vi "LCfiletrans(SubVI).vi"(8 "error in (no error)":errorcluster, 9 "Source Filename":string="D:\\Automation\\Data\\C1Title00030.csv", 11 "VISA Refnum in":refnum<visa-resource-name>="LecroyHDO4024-1") -> (0 "error out":errorcluster, 2 "File data":string, 3 "VISA Refnum out":refnum<visa-resource-name>)   [LabVIEW 2018]
uses:
  <instrlib>/LeCroy Wave Series/LeCroy Wave Series.lvlib
panel:
  in  "file path (use dialog)":path=path "E:/Ankur/Labview/Automation/Files/Oscdata/C1Title00030.csv"
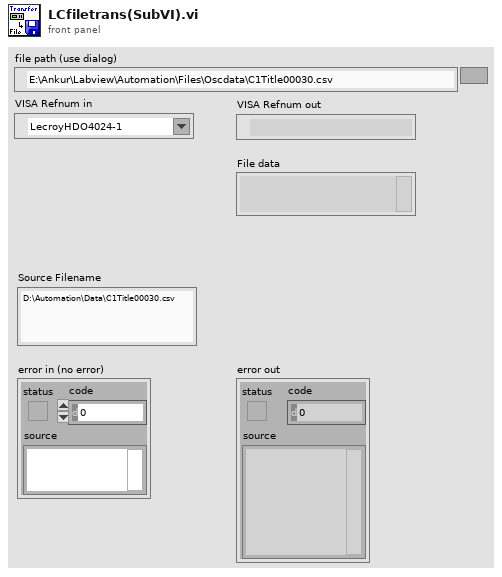
[diagram p1: front panel]
types:
  T1 = enum16{"open", "replace", "create", "open or create", "replace or create", "replace or create with confirmation"}
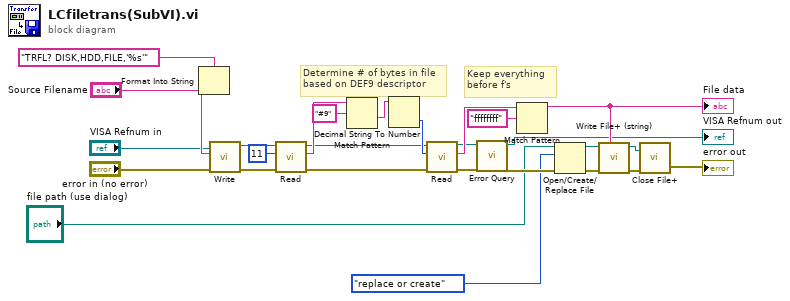
[diagram p0: block diagram]
diagram:
  # "Keep everything \nbefore f's"
  # "Determine # of bytes in file\nbased on DEF9 descriptor"
  n1 = Format Into String(format string="TRFL? DISK,HDD,FILE,'%s'" ("initial string"), "Source Filename") -> (resulting string=w7:string)  [unwired: 2 in, 1 out]
  n2 = call <instrlib>:"Write.vi"("error in (no error)"="error in (no error)", "Write Buffer"=w7, "VISA resource name"="VISA Refnum in") -> ("error out"=w11:errorcluster, "VISA resource name out"=w8:refnum<visa-resource-name>)  [unwired: 7 in]
  n3 = call <instrlib>:"Read.vi"("error in (no error)"=w11, "Byte Count"=u32 11, "VISA resource name"=w8) -> ("error out"=w12:errorcluster, "Read Buffer"=w14:string, "VISA resource name out"=w9:refnum<visa-resource-name>)  [unwired: 5 in, 1 out]
  n4 = Match Pattern(string=w14, regular expression="#9") -> (after substring=w16:string)  [unwired: 1 in, 3 out]
  n5 = Decimal String To Number(string=w16) -> (number=w17:i32)  [unwired: 2 in, 1 out]
  n6 = call <instrlib>:"Read.vi"("error in (no error)"=w12, "Byte Count"=w17, "VISA resource name"=w9) -> ("error out"=w22:errorcluster, "Read Buffer"=w19:string, "VISA resource name out"=w10:refnum<visa-resource-name>)  [unwired: 5 in, 1 out]
  n7 = call <instrlib>:"Error Query.vi"("error in (no error)"=w22, "VISA resource name"=w10) -> ("error out"=w23:errorcluster, "VISA resource name out"=→"VISA Refnum out":refnum<visa-resource-name>)  [unwired: 6 in, 2 out]
  n8 = Match Pattern(string=w19, regular expression="ffffffff") -> (before substring=w28:string)  [unwired: 1 in, 3 out]
  "File data" <- w28
  n9 = Open/Create/Replace File(file path (use dialog)="file path (use dialog)", error in=w23, operation (0:open)=T1."replace or create") -> (refnum out=w24:refnum<file>, error out=w20:errorcluster)  [unwired: 3 in, 1 out]
  n10 = call <vilib>:"Write File+ (string).vi"("string"=w28, "error in (no error)"=w20, "refnum"=w24) -> ("error out"=w21:errorcluster, "dup refnum"=w25:refnum<file>)  [unwired: 4 in, 1 out]
  n11 = call <vilib>:"Close File+.vi"("error in (no error)"=w21, "refnum"=w25) -> ("error out"=→"error out":errorcluster)  [unwired: 3 in, 2 out]
